vi "Convert Endpoint String to Endpoint.vi"(11 "Endpoint String":string) -> (3 "Endpoint":T1)   [LabVIEW 2019, in "Routing and Faulting System Explorer.lvlib"]
uses:
  Routing and Faulting System Explorer.lvlib
  Shared/Alias Endpoint.ctl
  Shared/Routing and Faulting Shared.lvlib
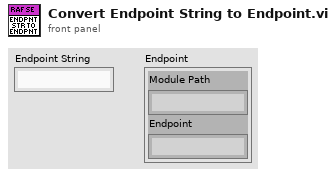
[diagram p1: front panel]
types:
  T1 = typedef "Routing and Faulting Shared.lvlib/Alias Endpoint.ctl" = cluster{"Module Path":string, "Endpoint":string}
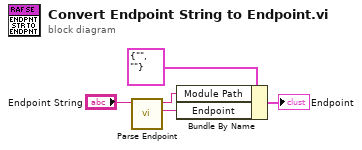
[diagram p0: block diagram]
diagram:
  n1 = call "Parse Endpoint.vi"("Module/Endpoint"="Endpoint String") -> ("Endpoint"=w1:string, "Module"=w2:string)  [unwired: 9 in]
  n2 = Bundle By Name(cluster=T1 {"Module Path"="", "Endpoint"=""} ("Endpoint"), "Module Path"=w2, "Endpoint"=w1) -> (→"Endpoint":T1)
